vi "LDA_data_rate.vi"() -> (1 "Data rate (Hz) BSA1":dbl format="%.1f", 2 "Data rate (Hz) BSA2":dbl format="%.1f")   [LabVIEW 2010]
uses:
  Controls/BSA_info_Cluster.ctl
  Globals/LDA_meas_global_1.vi
  Globals/LDA_meas_global_2.vi
panel:
  out "BSA2 info":T1={"GPIB Address"="13", "No of Check Bytes"=4, "Extra Info"="57N11", "COLOUR"=52224, "Wavelength (nm)"=52224.0} {"Wavelength (nm)" format="%.1f"}
  out "BSA1 info":T1={"GPIB Address"="13", "No of Check Bytes"=4, "Extra Info"="57N11", "COLOUR"=52224, "Wavelength (nm)"=52224.0} {"Wavelength (nm)" format="%.1f"}
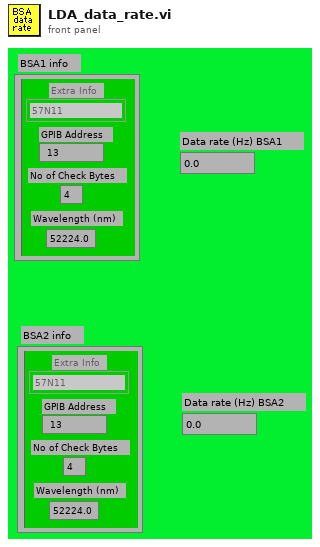
[diagram p1: front panel]
types:
  T1 = typedef "BSA_info_Cluster.ctl" = cluster{"GPIB Address":string, "No of Check Bytes":i32, "Extra Info":string, "COLOUR":u32, "Wavelength (nm)":dbl}
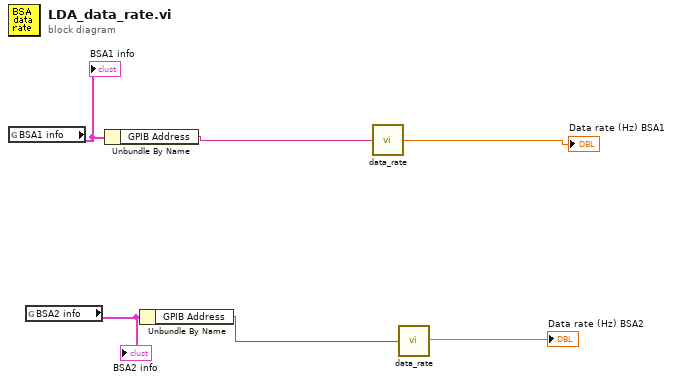
[diagram p0: block diagram]
diagram:
  n1 = global read "LDA_meas_global_1.vi" "BSA1 info"() -> (w6:T1)
  "BSA1 info" <- w6
  n2 = global read "LDA_meas_global_2.vi" "BSA2 info"() -> (w1:T1)
  "BSA2 info" <- w1
  n3 = Unbundle By Name(w6) -> ("GPIB Address"=w5:string)
  n4 = Unbundle By Name(w1) -> ("GPIB Address"=w2:string)
  n5 = call "data_rate.vi"("GPIB address"=w5) -> ("Data rate (Hz)"=→"Data rate (Hz) BSA1":dbl)
  n6 = call "data_rate.vi"("GPIB address"=w2) -> ("Data rate (Hz)"=→"Data rate (Hz) BSA2":dbl)
